vi "Status Update.vi"(7 "Command (Write)":T1, 8 "error in":errorcluster, 11 "Status Update":string) -> (0 "error out":errorcluster, 3 "queue out":refnum<queue>)   [LabVIEW 2018, in "Status Messaging.lvlib"]
uses:
  Status Messaging.lvlib
  Status Message Command.ctl
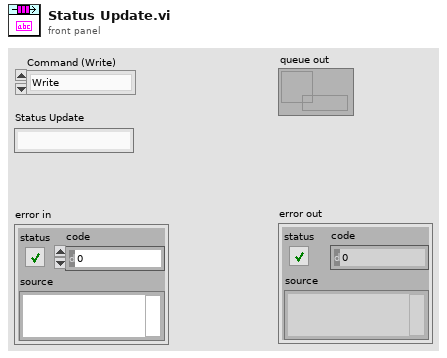
[diagram p1: front panel]
types:
  T1 = typedef "Status Messaging.lvlib/Status Message Command.ctl" = enum16{"Write", "Obtain", "Kill"}
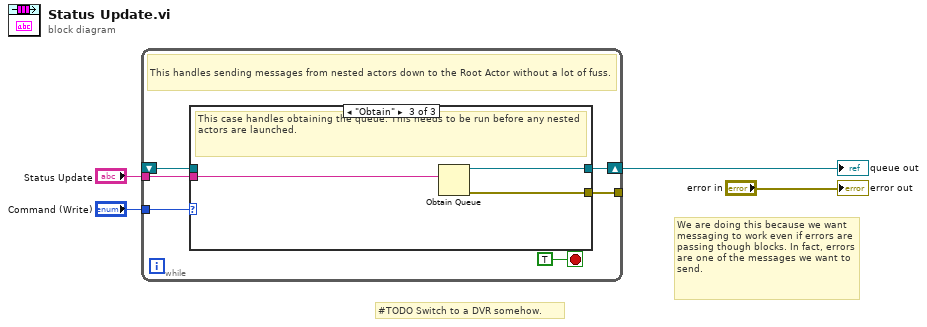
[diagram p0: block diagram]
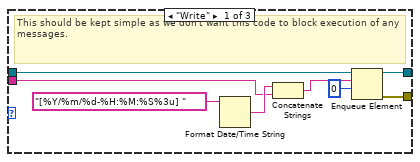
[diagram p2: hidden frame]
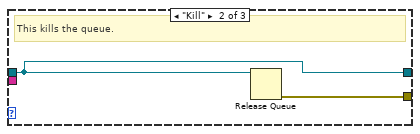
[diagram p3: hidden frame]
diagram:
  # "#TODO Switch to a DVR somehow."
  # "We are doing this because we want messaging to work even if errors are passing though blocks. In fact, errors are one of the messages we want to send."
  n1 = while {
    tunnel: "Command (Write)" -> [w9]
    tunnel: "Status Update" -> [w8]
    shift-right: [w7] -> w1
    shift-left: _ -> [w5]
    tunnel: [w6] -> _
    stop <- TRUE stop-if-true
    # "This handles sending messages from nested actors down to the Root Actor without a lot of fuss."
    n2 = case shown="\"Obtain\"" w9 {
      tunnel: w8 -> [w12 _ w21]
      tunnel: [w17 w19 w23] -> w7
      tunnel: [w16 w20 w22] -> w6
      tunnel: w5 -> [w18 w19 _]
      frame "Write" {
        # "This should be kept simple as we don't want this code to block execution of any messages."
        n3 = Format Date/Time String(time format string (%c)="[%Y/%m/%d-%H:%M:%S%3u] ") -> (date/time string=w13:string)  [unwired: 2 in]
        n4 = Concatenate Strings(w13, w12) -> (w11:string)
        n5 = Enqueue Element(queue=w18, element=w11, timeout in ms (-1)=0) -> (queue out=w17:refnum<queue>, error out=w16:errorcluster)  [unwired: 1 in, 1 out]
      }
      frame "Kill" {
        # "This kills the queue."
        n6 = Release Queue(queue=w19) -> (error out=w20:errorcluster)  [unwired: 2 in, 2 out]
      }
      frame "Obtain" {
        # "This case handles obtaining the queue. This needs to be run before any nested actors are launched."
        n7 = Obtain Queue(element data type=w21) -> (queue out=w23:refnum<queue>, error out=w22:errorcluster)  [unwired: 4 in, 1 out]
      }
    }
  }
  "queue out" <- w1
  "error out" <- "error in"
